vi "ReadSerial.vi"(9 "error in (no error)":errorcluster, 11 "VISA IN":refnum<visa-resource-name>) -> (0 "error out":errorcluster, 1 "bufferOut":string, 3 "VISA  OUT":refnum<visa-resource-name>)   [LabVIEW 2014]
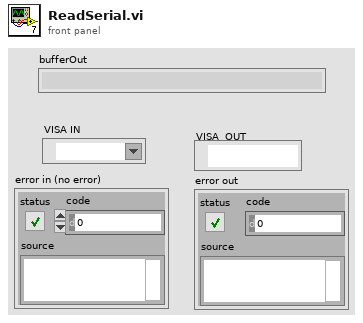
[diagram p1: front panel]
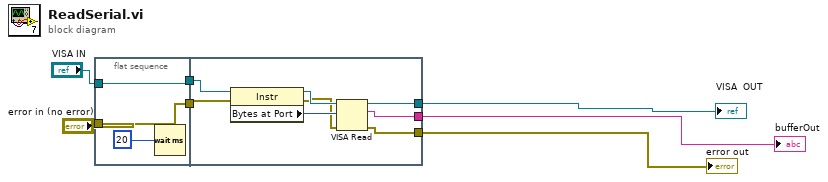
[diagram p0: block diagram]
diagram:
  n1 = flat-sequence {
    tunnel: "VISA IN" -> [w10]
    tunnel: "error in (no error)" -> [w9]
    tunnel: [w10] -> w5
    tunnel: [w9] -> w4
    tunnel: w5 -> [w18]
    tunnel: w4 -> [w14]
    tunnel: [w13] -> w3
    tunnel: [w12] -> w2
    tunnel: [w11] -> w1
    frame #0 {
      n2 = Wait (ms)(milliseconds to wait=u32 20 ("millisecond timer value")) -> ()  [unwired: 1 out]
    }
    frame #1 {
      n3 = property class="Instr"(reference=w18, error in=w14) -> (reference out=w17:refnum<visa-resource-name>, error out=w15:errorcluster, "Bytes at Port"=w16:u32)
      n4 = VISA Read(VISA resource name=w17, byte count=w16, error in (no error)=w15) -> (VISA resource name out=w12:refnum<visa-resource-name>, read buffer=w13:string, error out=w11:errorcluster)  [unwired: 1 out]
    }
  }
  "VISA  OUT" <- w2
  "error out" <- w1
  "bufferOut" <- w3
